vi "ExplorerTreeRecursiveFiles.vi"(4 "Folder to Exclude":string[](array[string]), 6 "Pattern":string, 8 "error in (no error)":errorcluster, 9 "Continue Recursing on Error? (F)":bool, 11 "Folder Path":path) -> (0 "error out":errorcluster, 1 "Folder Indexes":i32[](array[numeric]), 2 "Folders and Files":path[](array[path]), 3 "dup Folder Path":path)   [LabVIEW 2017]
doc: "List the content of a folder sorted by directories first. The <b>Folder Indexes</b> contain the index locations of the directories in the <b>Folders and Files</b> paths array. All other indexes are files.\n\nCreated By: Ryan Pacini"
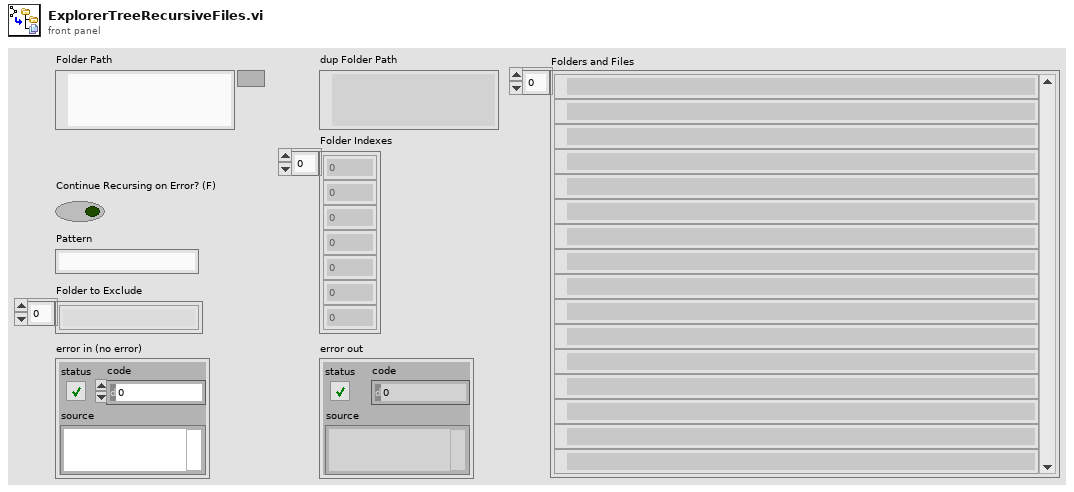
[diagram p1: front panel]
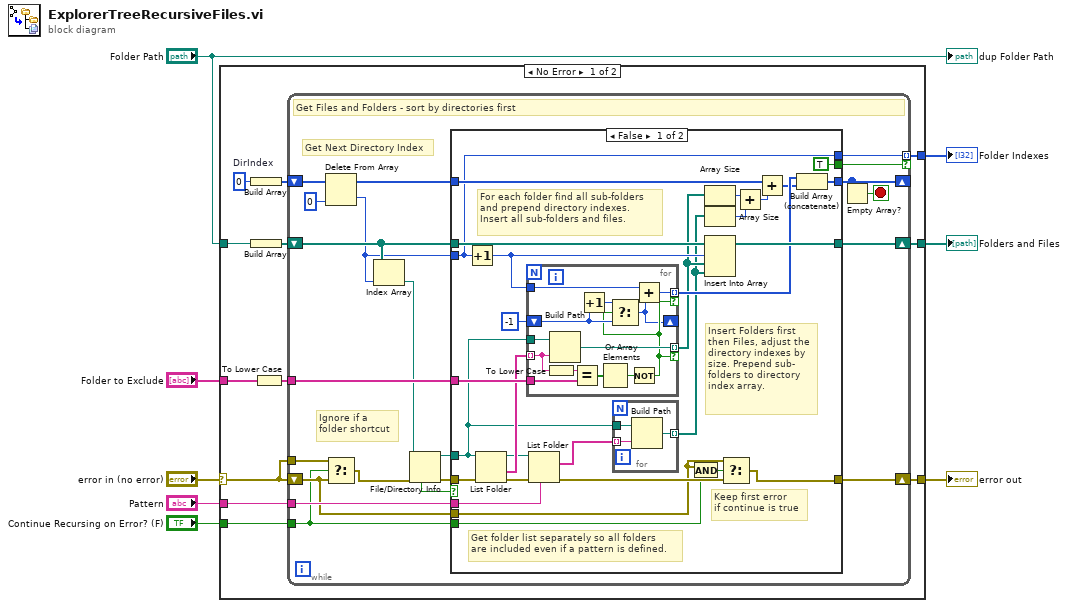
[diagram p0: block diagram]
diagram:
  n1 = case shown="No Error" "error in (no error)" {
    selector: "error in (no error)" -> [w11 w89]
    tunnel: "Folder to Exclude" -> [w20 _]
    tunnel: [w18 w89] -> w7
    tunnel: "Pattern" -> [w17 _]
    tunnel: [w13 _] -> w5
    tunnel: "Folder Path" -> [w12 _]
    tunnel: "Continue Recursing on Error? (F)" -> [w10 _]
    tunnel: [w9 _] -> w1
    frame No Error {
      w15 = 0  # DirIndex
      n2 = Build Array(w15) -> (w14:i32[])
      n3 = Build Array(w12) -> (w16:path[])
      n4 = To Lower Case(string=w20) -> (all lower case string=w19:string[])
      n5 = while {
        tunnel: w19 -> [w37]
        tunnel: w17 -> [w36]
        shift-right: [w35] -> w13
        shift-left: w16 -> [w34]
        shift-right: [w28] -> _
        shift-left: w14 -> [w32]
        shift-right: [w23] -> w18
        shift-left: w11 -> [w25]
        tunnel: w11 -> [w26]
        tunnel: w10 -> [w24]
        tunnel: [w22] -> w9 mode=indexing if=w21
        stop <- w38 stop-if-true
        # "Ignore if a\nfolder shortcut"
        # "Get Next Directory Index"
        # "Get Files and Folders - sort by directories first"
        n6 = Delete From Array(array=w32, index=0) -> (deleted portion=w31:i32, array with subset deleted=w29:i32[])  [unwired: 1 in]
        n7 = Select(t=w26, s=w24, f=w25) -> (s? t:f=w27:errorcluster)
        n8 = Index Array(array=w34, index=w31) -> (element=w33:path)
        n9 = File/Directory Info(path=w33, error in=w27) -> (path out=w40:path, error out=w41:errorcluster, shortcut=w39:bool)  [unwired: 4 out]
        n10 = case shown="False" w39 {
          tunnel: w41 -> [w69 w88]
          tunnel: w40 -> [w62 _]
          tunnel: [w48 w88] -> w23
          tunnel: w37 -> [w68 _]
          tunnel: [w61 w87] -> w35
          tunnel: w36 -> [w63 _]
          tunnel: w34 -> [w60 w87]
          tunnel: w31 -> [w44 _]
          tunnel: w29 -> [w51 w86]
          tunnel: [w57 w86] -> w28
          tunnel: w25 -> [w46 _]
          tunnel: w24 -> [w47 _]
          tunnel: [w44 _] -> w22
          tunnel: [TRUE _] -> w21
          frame False {
            # "Keep first error\nif continue is true"
            # "Get folder list separately so all folders \nare included even if a pattern is defined."
            # "For each folder find all sub-folders\nand prepend directory indexes.\nInsert all sub-folders and files."
            # "Insert Folders first\nthen Files, adjust the\ndirectory indexes by\nsize. Prepend sub-\nfolders to directory\nindex array."
            n11 = Increment(x=w44) -> (x+1=w59:i32)
            n12 = List Folder(path=w62, error in=w69) -> (path out=w64:path, folder names=w67:string[], error out=w65:errorcluster)  [unwired: 2 in, 1 out]
            n13 = for {
              tunnel: w67 -> [w80] mode=indexing
              tunnel: w62 -> [w85]
              tunnel: w68 -> [w83]
              tunnel: [w79] -> w56 mode=indexing if=w74
              tunnel: w59 -> [w78]
              tunnel: [w77] -> w58 mode=indexing if=w74
              shift-right: [w73] -> _
              shift-left: -1 -> [w75]
              # "Exclude Folders"
              n14 = To Lower Case(string=w80) -> (all lower case string=w84:string)
              n15 = Build Path(base path=w85, name or relative path=w80) -> (appended path=w79:path)
              n16 = Equal?(x=w84, y=w83) -> (x = y?=w82:bool[])
              n17 = Increment(x=w75) -> (x+1=w76:i32)
              n18 = Or Array Elements(Boolean array=w82) -> (logical OR=w81:bool)
              n19 = Not(x=w81) -> (.not. x?=w74:bool)
              n20 = Select(t=w76, s=w74, f=w75) -> (s? t:f=w73:i32)
              n21 = Add(x=w78, y=w73) -> (x+y=w77:i32)
            }
            n22 = List Folder(path=w64, pattern=w63, error in=w65) -> (filenames=w66:string[], error out=w49:errorcluster)  [unwired: 1 in, 2 out]
            n23 = for {
              tunnel: w62 -> [w72]
              tunnel: w66 -> [w71] mode=indexing
              tunnel: [w70] -> w55 mode=indexing
              n24 = Build Path(base path=w72, name or relative path=w71) -> (appended path=w70:path)
            }
            n25 = And(x=w46, y=w47) -> (x .and. y?=w45:bool)
            n26 = Array Size(array=w56) -> (size(s)=w54:i32)
            n27 = Array Size(array=w55) -> (size(s)=w53:i32)
            n28 = Insert Into Array(array=w60, index=w59, new element #1=w56, new element #2=w55) -> (w61:path[])
            n29 = Select(t=w46, s=w45, f=w49) -> (s? t:f=w48:errorcluster)
            n30 = Add(x=w54, y=w53) -> (x+y=w52:i32)
            n31 = Add(x=w51, y=w52) -> (x+y=w50:i32[])
            n32 = Build Array (concatenate)(w58, w50) -> (w57:i32[])
          }
          frame True {
            # "Directory is a shortcut, do nothing"
          }
        }
        n33 = Empty Array?(array=w28) -> (empty?=w38:bool)
      }
    }
    frame Error {
    }
  }
  "error out" <- w7
  "Folders and Files" <- w5
  "Folder Indexes" <- w1
  "dup Folder Path" <- "Folder Path"
